vi "Bootloader - Write Page.vi"(0 "VISA resource name":refnum<visa-resource-name>, 5 "Address":u32, 7 "Data Length":u32, 9 "Data":u8[](array[numeric]), 11 "error in (no error)":errorcluster) -> (4 "VISA resource name":refnum<visa-resource-name>, 6 "Address":u32, 8 "Data Length":u32, 10 "Data":u8[](array[numeric]), 15 "error out":errorcluster)   [LabVIEW 2010]
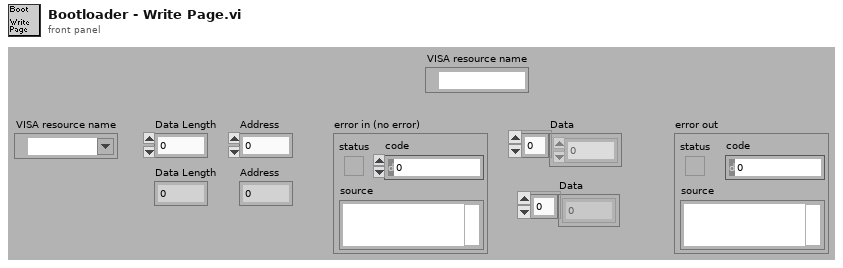
[diagram p1: front panel]
types:
  T1 = enum16{"big-endian, network order", "native, host order", "little-endian"}
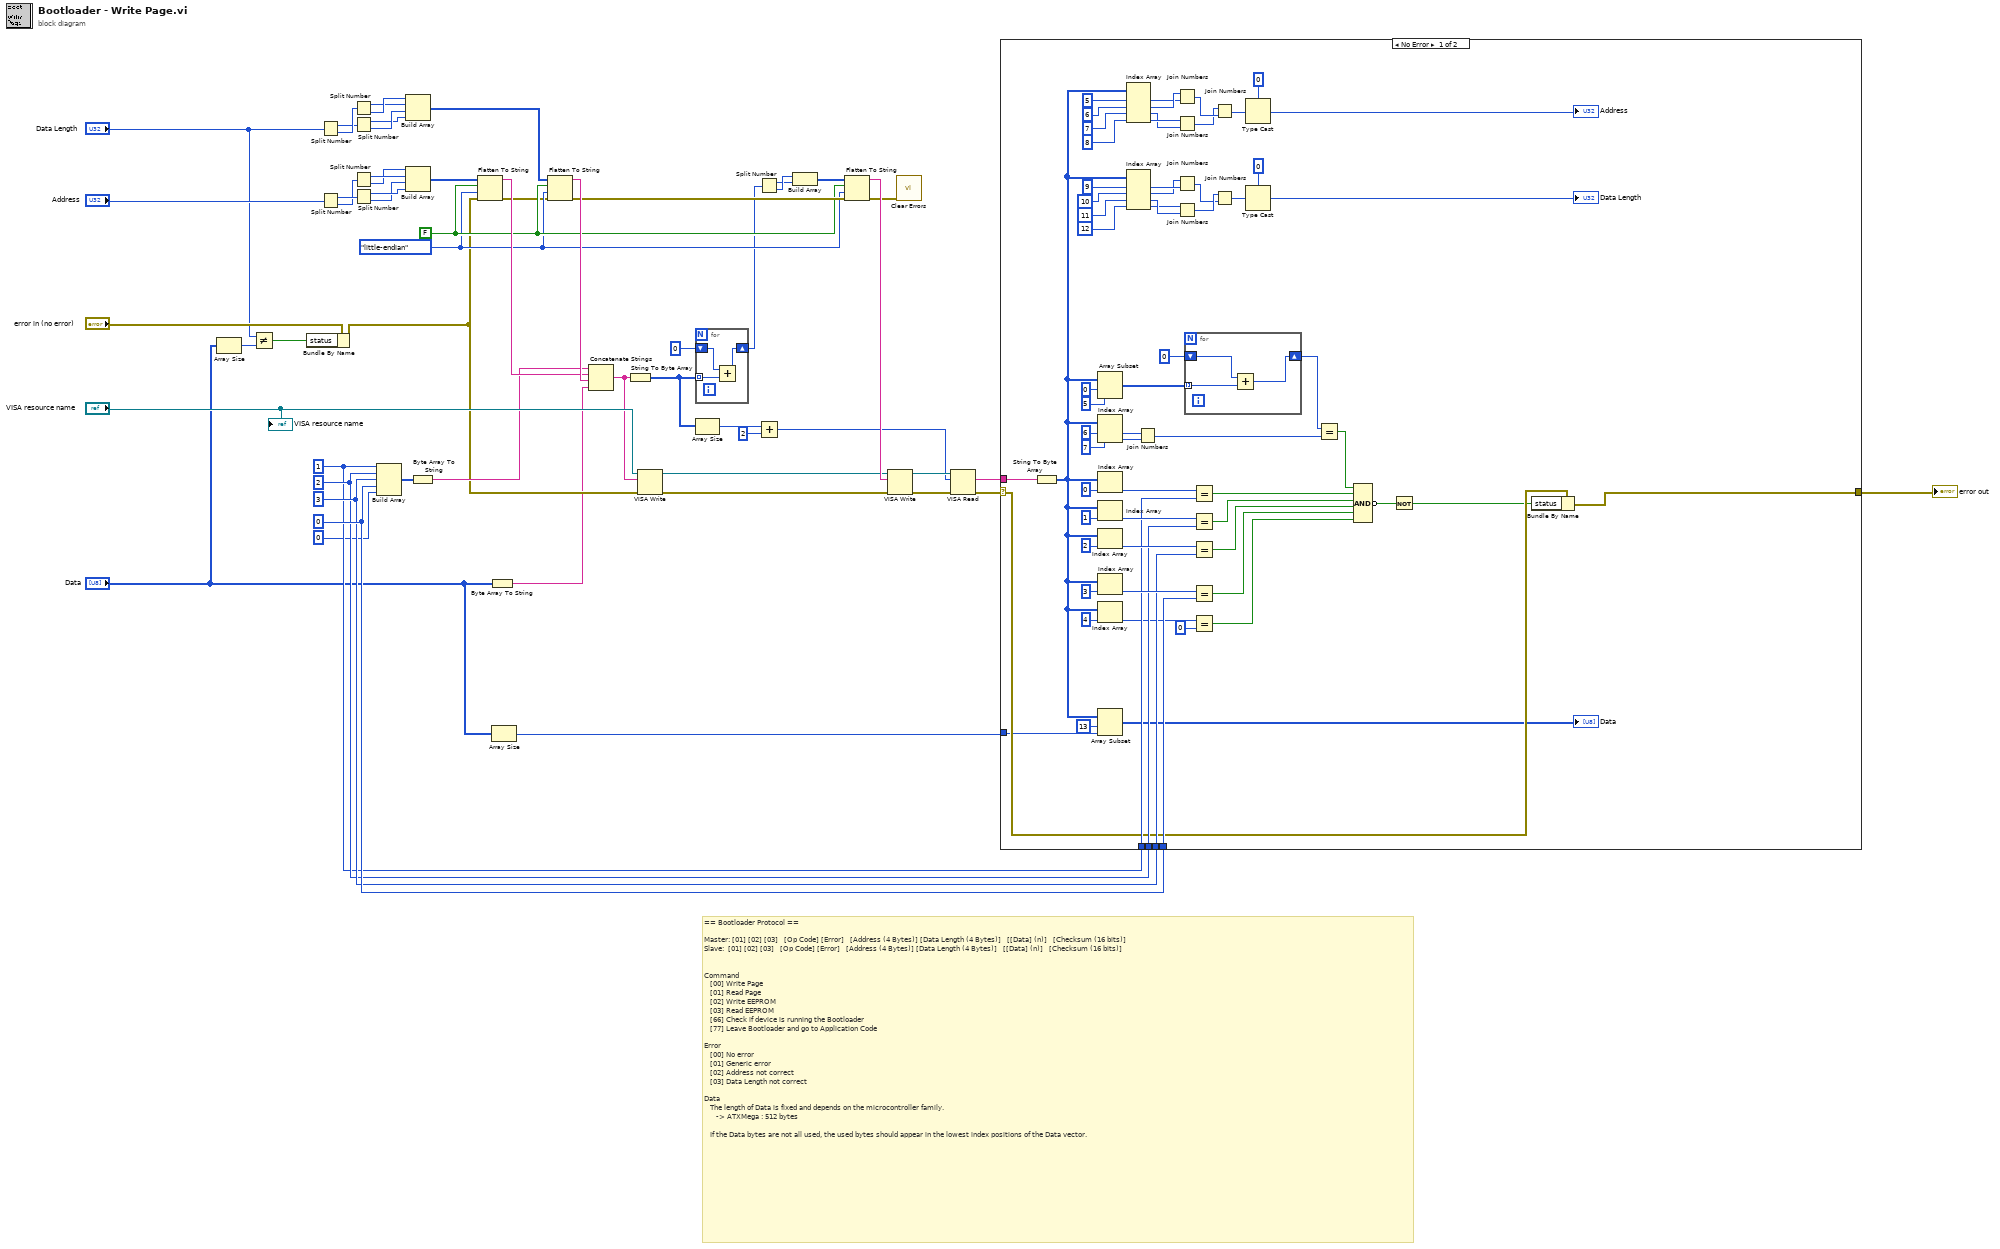
[diagram p0: block diagram]
diagram:
  w36 = T1."little-endian" ("byte order (0:big-endian, network order)")
  w37 = FALSE ("prepend array or string size? (T)")
  w47 = u8 0 ("element")
  w46 = u8 3 ("element")
  w45 = u8 2 ("element")
  w44 = u8 1 ("element")
  # "== Bootloader Protocol ==\n\nMaster: [01] [02] [03]   [Op Code] [Error]   [Address (4 Bytes)] [Data Length (4 Bytes)]   [[Data] (n)]   [Checksum (16 bits)]\nSlave:  [01] [02] [03]   [Op Code] [Error]   [Address (4 Bytes)] [Data Length (4 Bytes)]   [[Data] (n)]   [Checksum (16 bits)]\n\n\nCommand\n   [00] Write Page\n   [01] Read Page\n   [02] Write EEPROM\n   [03] Read EEPROM\n   [66] Check if device is running the Bootloader\n   [77] Leave Bootloader and go to Application Code\n\nError\n   [00] No error\n   [01] Generic error\n   [02] Address not correct\n   [03] Data Length not correct\n\nData\n   The length of Data is fixed and depends on the microcontroller family.\n      -> ATXMega : 512 bytes\n\n   If the Data bytes are not all used, the used bytes should appear in the lowest index positions of the Data vector."
  n1 = Array Size(array="Data") -> (size(s)=w13:i32)
  n2 = Not Equal?(x="Data Length", y=w13) -> (x != y?=w10:bool)
  n3 = Bundle By Name(cluster="error in (no error)", "status"=w10) -> (w11:errorcluster)
  n4 = Split Number(x="Data Length") -> (hi(x)=w23:u16, lo(x)=w24:u16)
  n5 = Split Number(x="Address") -> (hi(x)=w18:u16, lo(x)=w17:u16)
  n6 = Split Number(x=w24) -> (hi(x)=w25:u8, lo(x)=w26:u8)
  n7 = Split Number(x=w23) -> (hi(x)=w21:u8, lo(x)=w22:u8)
  n8 = Split Number(x=w17) -> (hi(x)=w16:u8, lo(x)=w15:u8)
  n9 = Split Number(x=w18) -> (hi(x)=w20:u8, lo(x)=w19:u8)
  n10 = Build Array(w44, w45, w46, w47, u8 0 ("element")) -> (w30:u8[])
  n11 = Build Array(w26, w25, w22, w21) -> (w28:u8[])
  n12 = Build Array(w15, w16, w19, w20) -> (w14:u8[])
  n13 = Byte Array To String(unsigned byte array=w30) -> (string=w48:string)
  n14 = Flatten To String(anything=w14, prepend array or string size? (T)=w37, byte order (0:big-endian, network order)=w36, error in (no error)=w11) -> (data string=w49:string, error out=w27:errorcluster)  [unwired: 1 out]
  n15 = Byte Array To String(unsigned byte array="Data") -> (string=w8:string)
  n16 = Array Size(array="Data") -> (size(s)=w1:i32)
  n17 = Flatten To String(anything=w28, prepend array or string size? (T)=w37, byte order (0:big-endian, network order)=w36, error in (no error)=w27) -> (data string=w50:string, error out=w38:errorcluster)  [unwired: 1 out]
  n18 = Concatenate Strings(w48, w49, w50, w8) -> (w51:string)
  n19 = String To Byte Array(string=w51) -> (unsigned byte array=w9:u8[])
  n20 = VISA Write(VISA resource name="VISA resource name", write buffer=w51, error in (no error)=w11) -> (VISA resource name out=w7:refnum<visa-resource-name>, error out=w6:errorcluster)  [unwired: 1 out]
  n21 = Array Size(array=w9) -> (size(s)=w5:i32)
  n22 = for {
    tunnel: w9 -> [w59] mode=indexing
    shift-right: [w57] -> w35
    shift-left: u16 0 ("page address") -> [w58]
    n23 = Add(x=w58, y=w59) -> (x+y=w57:u16)
  }
  n24 = Split Number(x=w35) -> (hi(x)=w32:u8, lo(x)=w33:u8)
  n25 = Add(x=w5, y=2) -> (x+y=w3:i32)
  n26 = Build Array(w33, w32) -> (w34:u8[])
  n27 = Flatten To String(anything=w34, prepend array or string size? (T)=w37, byte order (0:big-endian, network order)=w36, error in (no error)=w38) -> (data string=w40:string, error out=w39:errorcluster)  [unwired: 1 out]
  n28 = VISA Write(VISA resource name=w7, write buffer=w40, error in (no error)=w6) -> (VISA resource name out=w42:refnum<visa-resource-name>, error out=w41:errorcluster)  [unwired: 1 out]
  n29 = call <vilib>:"Clear Errors.vi"("error in (no error)"=w39) -> ()  [unwired: 6 in, 1 out]
  n30 = VISA Read(VISA resource name=w42, byte count=w3, error in (no error)=w41) -> (read buffer=w43:string, error out=w53:errorcluster)  [unwired: 2 out]
  n31 = case shown="No Error" w53 {
    selector: w53 -> [w92 w129]
    tunnel: w43 -> [w125 _]
    tunnel: w44 -> [w115 _]
    tunnel: w45 -> [w114 _]
    tunnel: w46 -> [w113 _]
    tunnel: w47 -> [w112 _]
    tunnel: [w91 w129] -> w54
    tunnel: w1 -> [w61 _]
    frame No Error {
      n32 = String To Byte Array(string=w125) -> (unsigned byte array=w62:u8[])
      n33 = Array Subset(array=w62, index=0, length=5) -> (w101:u8[])
      n34 = Index Array(array=w62, index #1=6 ("index"), index #2=7 ("index")) -> (element #1=w98:u8, element #2=w97:u8)
      n35 = Index Array(array=w62, index=0) -> (element=w119:u8)
      n36 = Index Array(array=w62, index=1) -> (element=w118:u8)
      n37 = Index Array(array=w62, index=2) -> (element=w117:u8)
      n38 = Index Array(array=w62, index=3) -> (element=w116:u8)
      n39 = Index Array(array=w62, index=4) -> (element=w107:u8)
      n40 = Array Subset(array=w62, index=13, length=w61) -> (→"Data":u8[])
      n41 = Index Array(array=w62, index #1=5 ("index"), index #2=6 ("index"), index #3=7 ("index"), index #4=8 ("index")) -> (element #1=w82:u8, element #2=w86:u8, element #3=w83:u8, element #4=w84:u8)
      n42 = Index Array(array=w62, index #1=9 ("index"), index #2=10 ("index"), index #3=11 ("index"), index #4=12 ("index")) -> (element #1=w73:u8, element #2=w69:u8, element #3=w72:u8, element #4=w71:u8)
      n43 = Join Numbers(hi=w98, lo=w97) -> ((hi.lo)=w96:u16)
      n44 = Join Numbers(hi=w86, lo=w82) -> ((hi.lo)=w87:u16)
      n45 = Join Numbers(hi=w84, lo=w83) -> ((hi.lo)=w85:u16)
      n46 = Join Numbers(hi=w69, lo=w73) -> ((hi.lo)=w68:u16)
      n47 = Join Numbers(hi=w71, lo=w72) -> ((hi.lo)=w70:u16)
      n48 = for {
        tunnel: w101 -> [w128] mode=indexing
        shift-right: [w126] -> w95
        shift-left: u16 0 ("page address") -> [w127]
        n49 = Add(x=w127, y=w128) -> (x+y=w126:u16)
      }
      n50 = Equal?(x=w119, y=w115) -> (x = y?=w111:bool)
      n51 = Equal?(x=w118, y=w114) -> (x = y?=w110:bool)
      n52 = Equal?(x=w117, y=w113) -> (x = y?=w109:bool)
      n53 = Equal?(x=w116, y=w112) -> (x = y?=w108:bool)
      n54 = Equal?(x=w107, y=u8 0) -> (x = y?=w105:bool)
      n55 = Join Numbers(hi=w85, lo=w87) -> ((hi.lo)=w88:u32)
      n56 = Join Numbers(hi=w70, lo=w68) -> ((hi.lo)=w67:u32)
      n57 = Type Cast(type=u32 0 ("byte count"), x=w88) -> (*(type *) &x=→"Address":u32)
      n58 = Type Cast(type=u32 0 ("byte count"), x=w67) -> (*(type *) &x=→"Data Length":u32)
      n59 = Equal?(x=w95, y=w96) -> (x = y?=w94:bool)
      n60 = Compound Arithmetic op=AND(w94, w111, w110, w109, w108, w105) -> (invert w93:bool)
      n61 = Not(x=w93) -> (.not. x?=w90:bool)
      n62 = Bundle By Name(cluster=w92, "status"=w90) -> (w91:errorcluster)
    }
    frame Error {
    }
  }
  "error out" <- w54
  "VISA resource name" <- "VISA resource name"
